vi "Check Active Grape Effect.vi"(8 "error in (no error)":errorcluster, 10 "Packed refs":T1, 11 "Grape in":refnum<class "Grape.lvclass">) -> (0 "error out":errorcluster, 2 "Still Active?":bool, 3 "Grape out":refnum<class "Grape.lvclass">)   [LabVIEW 2021, in "Grape.lvclass"]
uses:
  Grape.lvclass
  Application/Packed Refs.ctl
  GameEl_class/private/Enum Direction.ctl
  Grape.lvclass/Grape.ctl
  Imposible_Snake_v2/LVApp/Modules/Sound Manager/Typedefs/Sound Effects.ctl
  <vilib>/numeric/Random Number (Range) DBL.vi
  Imposible_Snake_v2/LVApp/Modules/Sound Manager/Sound Manager.lvlib
  GameEl_class/GameEl.lvclass
  Application/Game.lvclass
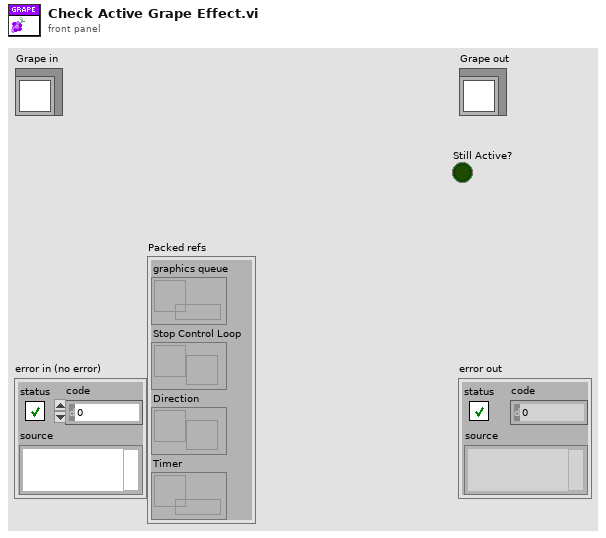
[diagram p1: front panel]
types:
  T1 = typedef "Game.lvclass/Packed Refs.ctl" = cluster{"graphics queue":refnum<queue>, "Stop Control Loop":refnum<user-event>, "Direction":refnum<notifier>, "Timer":refnum<data-value>}
  T2 = typedef "Sound Manager.lvlib/Sound Effects.ctl" = enum16{"Bomb In", "Bomb Out", "Bomb Touched", "Game Over", "Victory", "Eat", "10 Fruits", "Eat2", "Eat3", "Eat4", "MaxShield", "Shield", "10p", "Grape In", "Grape Out", "20p", "30p", "40p", "50p", "60p", "70p", "80p", "90p", "100p", "All shields cracked", "Mouse In", "Mouse Out", "Mouse Eaten", "Grape Eaten", "States Recover", "Broken Shield", "Bonus", "Happy Time", "explode", "Game over musica", "Back Music", "Shield Catch", "Evil lough", "Cricket In", "Cricket eaten", "Lets Go", "Jump1", "Jump2", "Jump3", "Unstoppable", "Troll Music", "winner", "menu"}
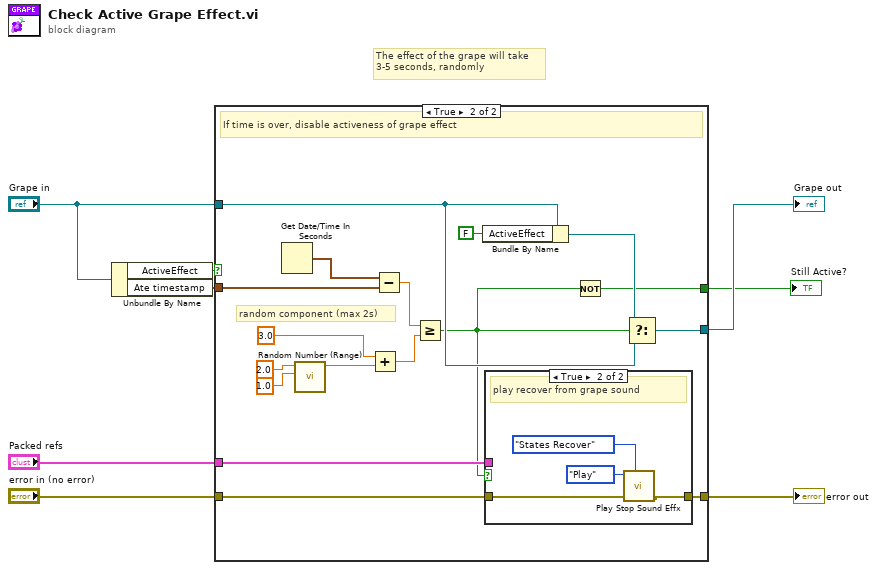
[diagram p0: block diagram]
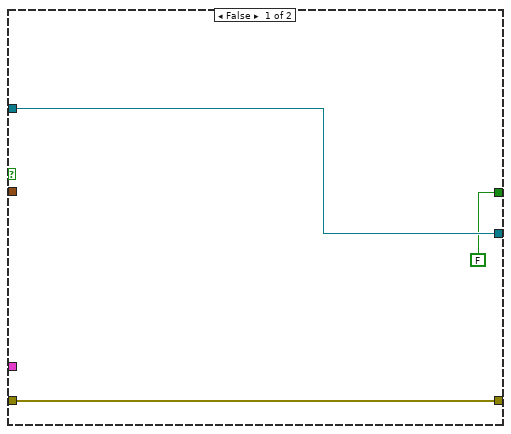
[diagram p2: hidden frame]
diagram:
  # "The effect of the grape will take \n3-5 seconds, randomly"
  n1 = Unbundle By Name("Grape in") -> ("ActiveEffect"=w8:bool, "Ate timestamp"=w7:timestamp)
  n2 = case shown="True" w8 {
    tunnel: w7 -> [_ w27]
    tunnel: "Grape in" -> [w11 w18]
    tunnel: [w11 w17] -> w5
    tunnel: [FALSE w16] -> w4
    tunnel: "error in (no error)" -> [w9 w15]
    tunnel: [w9 w14] -> w2
    tunnel: "Packed refs" -> [_ w13]
    frame False {
    }
    frame True {
      # "random component (max 2s)"
      # "If time is over, disable activeness of grape effect"
      n3 = Get Date/Time In Seconds() -> (seconds since 1Jan1904=w28:timestamp)
      n4 = call-poly <vilib>:"Random Number (Range).vi"("lower bound (0)"=1.0 ("Low"), "upper bound (100)"=2.0 ("High")) -> ("number"=w22:dbl)  [unwired: 9 in]
      n5 = Add(x=3.0 ("y"), y=w22) -> (x+y=w21:dbl)
      n6 = Subtract(x=w28, y=w27) -> (x-y=w26:dbl)
      n7 = Greater Or Equal?(x=w26, y=w21) -> (x >= y?=w12:bool)
      n8 = Bundle By Name(cluster=w18, "ActiveEffect"=FALSE) -> (w19:refnum<class "Grape.lvclass">)
      n9 = case shown="True" w12 {
        tunnel: w15 -> [w29 w31]
        tunnel: [w29 w30] -> w14
        tunnel: w13 -> [_ _]
        frame False {
        }
        frame True {
          # "play recover from grape sound"
          n10 = call "Play Stop Sound Effx.vi"("Sound Effect"=Sound_Effects."States Recover", "Error In"=w31, "Function"=enum16{"Play", "Stop"}."Play") -> ("error in (no error)"=w30:errorcluster)  [unwired: 8 in]
        }
      }
      n11 = Not(x=w12) -> (.not. x?=w16:bool)
      n12 = Select(t=w19, s=w12, f=w18) -> (s? t:f=w17:refnum<class "Grape.lvclass">)
    }
  }
  "error out" <- w2
  "Grape out" <- w5
  "Still Active?" <- w4
